vi "Save Configuration.vi"(7 "Slave Address":i32=-1 min=-1 max=30 step=1, 8 "error":errorcluster, 11 "VISA":refnum<visa-resource-name>) -> (0 "error out":errorcluster, 3 "VISA out":refnum<visa-resource-name>)   [LabVIEW 2025, in "TDK-Lambda GEN LAN Series.lvlib"]
doc: "Saves the power supply settings so they may be recalled at a later time. The settings which are saved are the same as the power-up settings. They include:\n\n- Output On/Off - Over-Voltage Setting \n- Programmed Voltage - Programmed Current \n- Under-Voltage Setting - Lock Front Panel\n- Fold-back Enabled or not - Auto-Start or Safe-Start\n\nThe saved settings are lost when the unit is powered down"
uses:
  <userlib>/TDK-Lambda GEN LAN Series/TDK-Lambda GEN LAN Series.lvlib
panel:
  # "TDK-Lambda Genesys \n LAN\n  DC Power Supplies"
  # "Save Instrument Setup"
  # "(c) 2019 TDK-Lambda.  ALL RIGHTS RESERVED."
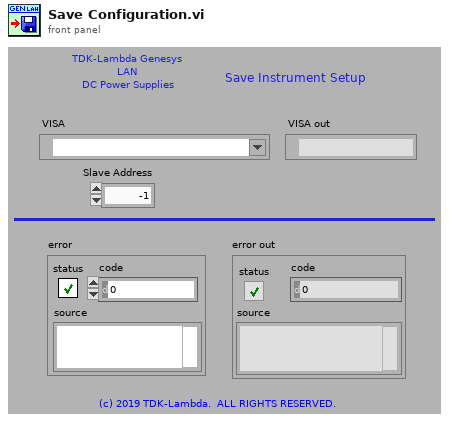
[diagram p1: front panel]
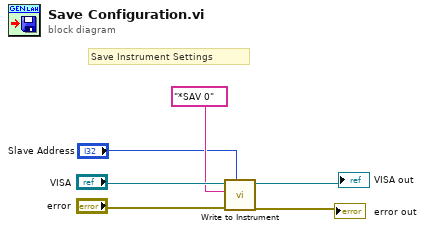
[diagram p0: block diagram]
diagram:
  # "Save Instrument Settings"
  n1 = call <userlib>:"Write to Instrument.vi"("Slave Address"="Slave Address", "error"="error", "Command"="*SAV 0" ("format string"), "VISA"="VISA") -> ("error out"=→"error out":errorcluster, "VISA out"=→"VISA out":refnum<visa-resource-name>)  [unwired: 6 in]
